vi "z did wid and eid.vi"(0 "Device In":T1, 5 "did":string, 7 "wid":string, 9 "eid":string, 11 "error in":errorcluster) -> (4 "Device Out":T1, 15 "error out":errorcluster)   [LabVIEW 2021]
uses:
  Cluster.ctl
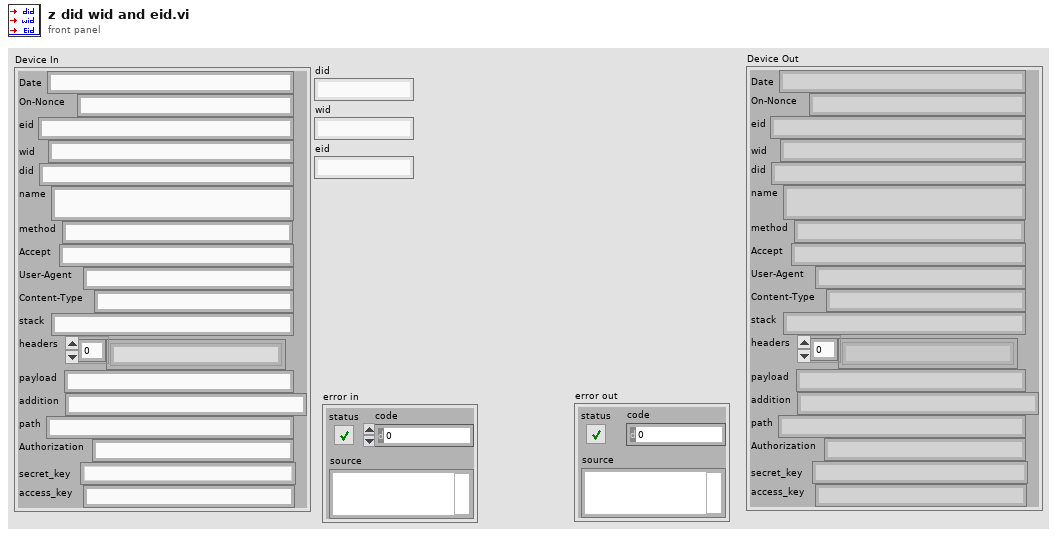
[diagram p1: front panel]
types:
  T1 = typedef "Cluster.ctl" = cluster{"Date":string, "On-Nonce":string, "eid":string, "wid":string, "did":string, "name":string, "method":string, "Accept":string, "User-Agent":string, "Content-Type":string, "stack":string, "headers":string[], "payload":string, "addition":string, "path":string, "Authorization":string, "secret_key":string, "access_key":string}
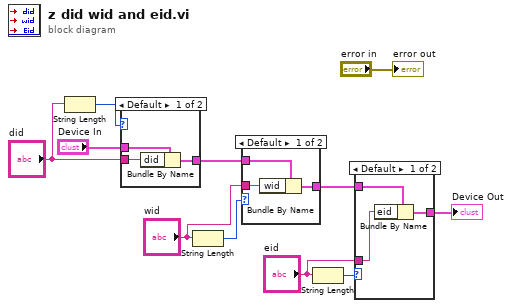
[diagram p0: block diagram]
diagram:
  n1 = String Length(string="did") -> (length=w10:i32)
  n2 = case shown="Default" w10 {
    tunnel: "Device In" -> [w14 w15]
    tunnel: [w12 w15] -> w4
    tunnel: "did" -> [w13 _]
    frame Default {
      n3 = Bundle By Name(cluster=w14, "did"=w13) -> (w12:T1)
    }
    frame 0 {
    }
  }
  n4 = String Length(string="wid") -> (length=w7:i32)
  n5 = case shown="Default" w7 {
    tunnel: w4 -> [w18 w19]
    tunnel: [w16 w19] -> w2
    tunnel: "wid" -> [w17 _]
    frame Default {
      n6 = Bundle By Name(cluster=w18, "wid"=w17) -> (w16:T1)
    }
    frame 0 {
    }
  }
  n7 = String Length(string="eid") -> (length=w6:i32)
  n8 = case shown="Default" w6 {
    tunnel: w2 -> [w22 w23]
    tunnel: [w20 w23] -> w1
    tunnel: "eid" -> [w21 _]
    frame Default {
      n9 = Bundle By Name(cluster=w22, "eid"=w21) -> (w20:T1)
    }
    frame 0 {
    }
  }
  "Device Out" <- w1
  "error out" <- "error in"
